vi "Main.vi"(11 "Script in":refnum<class "_Template.lvclass">) -> ()   [LabVIEW 2021, in "_Template.lvlib" / "_Template.lvclass"]
uses:
  _Template.lvclass
  _Template.lvclass/_Template.ctl
  _Rename/_Rename/_Rename.lvclass
  _Shared/_Shared.lvlib
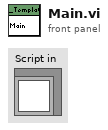
[diagram p1: front panel]
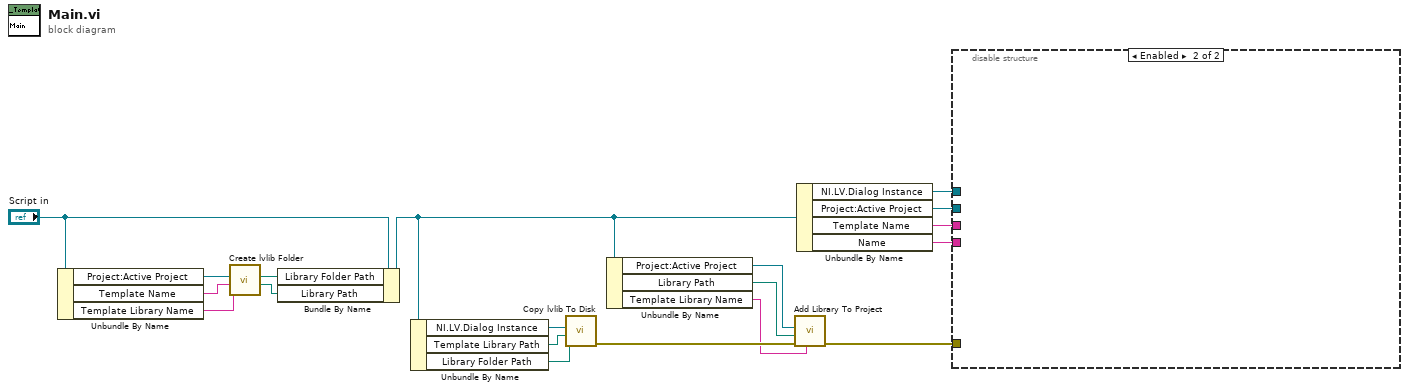
[diagram p0: block diagram]
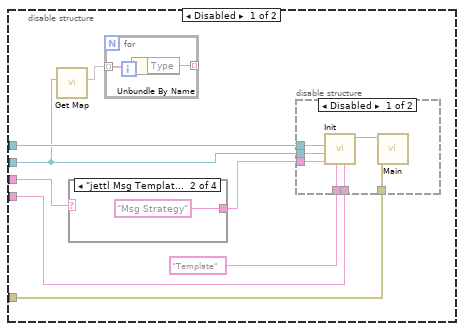
[diagram p2: hidden frame]
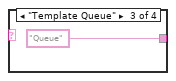
[diagram p5: hidden frame]
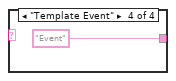
[diagram p6: hidden frame]
diagram:
  n1 = Unbundle By Name("Script in") -> ("Project:Active Project"=w19:refnum<vi>, "Template Name"=w9:string, "Template Library Name"=w8:string)
  n2 = call "Create lvlib Folder.vi"("Template Library Name"=w8, "Template Name"=w9, "Project:Active Project"=w19) -> ("Library Path"=w11:path, "Library Folder Path"=w18:path)  [unwired: 7 in]
  n3 = Bundle By Name(cluster="Script in", "Library Folder Path"=w18, "Library Path"=w11) -> (w6:refnum<class "_Template.lvclass">)
  n4 = Unbundle By Name(w6) -> ("NI.LV.Dialog Instance"=w16:refnum<vi>, "Template Library Path"=w15:path, "Library Folder Path"=w14:path)
  n5 = call "Copy lvlib To Disk.vi"("Library Folder Path"=w14, "Template Library Path"=w15, "NI.LV.Dialog Instance"=w16) -> ("error out"=w13:errorcluster)  [unwired: 8 in]
  n6 = Unbundle By Name(w6) -> ("Project:Active Project"=w17:refnum<vi>, "Library Path"=w10:path, "Template Library Name"=w7:string)
  n7 = call "Add Library To Project.vi"("Template Library Name"=w7, "error in"=w13, "Library Path"=w10, "Project:Active Project"=w17) -> ("error out"=w4:errorcluster)  [unwired: 7 in]
  n8 = Unbundle By Name(w6) -> ("NI.LV.Dialog Instance"=w3:refnum<vi>, "Project:Active Project"=w1:refnum<vi>, "Template Name"=w5:string, "Name"=w2:string)
  n9 = disable-structure shown="Enabled" {
    disable-tunnel: w5 -> [w27 _]
    disable-tunnel: w4 -> [w25 _]
    disable-tunnel: w3 -> [w24 _]
    disable-tunnel: w2 -> [w22 _]
    disable-tunnel: w1 -> [w21 _]
    frame Disabled {
      n10 = call "Get Map.vi"("Project:Active Project"=w21) -> ("Type Name Path"=w20:map{string, map{string, path}})  [unwired: 10 in]
      n11 = case shown="\"jettl Msg Template\"" w27 {
        tunnel: [_ "Msg Strategy" ("Template Name") "Queue" ("Template Name") "Event" ("Template Name")] -> w26
        frame Default {
        }
        frame "jettl Msg Template" {
        }
        frame "Template Queue" {
        }
        frame "Template Event" {
        }
      }
      n12 = for {
        tunnel: w20 -> [w29] mode=indexing
        tunnel: [w28] -> _ mode=indexing
        n13 = Unbundle By Name(w29) -> ("Type"=w28:string)
      }
      n14 = disable-structure shown="Disabled" {
        disable-tunnel: w26 -> [w36 _]
        disable-tunnel: w25 -> [w34 _]
        disable-tunnel: w24 -> [w33 _]
        disable-tunnel: w21 -> [w32 _]
        disable-tunnel: "Template" ("Name") -> [w31 _]
        disable-tunnel: w22 -> [w30 _]
        frame Disabled {
          n15 = call "Init.vi"("Rename"=w30, "Name"=w31, "Type"=w36, "Project:Active Project"=w32, "NI.LV.Dialog Instance"=w33) -> ("Script out"=w35:refnum<class "_Rename.lvclass">)  [unwired: 6 in]
          n16 = call "Main.vi"("error in"=w34, "Script in"=w35) -> ()  [unwired: 10 in]
        }
        frame Enabled {
        }
      }
    }
    frame Enabled {
    }
  }
